vi "PXIe 4113 Config.vi"(8 "error in (no error)":errorcluster, 11 "Device Ref in":T1 format="%.0x") -> (0 "error out":errorcluster, 2 "instrument handle out":refnum<k15>, 3 "Device Ref out":T1 format="%.0x")   [LabVIEW 2015, in "PXIe 4113 Engine.lvlib"]
uses:
  PXIe 4113 Engine.lvlib
  <vilib>/NI Veristand/Custom Device API/Custom Device Item Ref.ctl
  <instrlib>/niDCPower/nidcpower.llb/niDCPower Source Mode.ctl
  <instrlib>/niDCPower/nidcpower.llb/niDCPower Output Function.ctl
  <instrlib>/niDCPower/nidcpower.llb/niDCPower Sense.ctl
  Shared/Constants.vi
  <vilib>/NI Veristand/Custom Device API/Get Item Property (String).vi
  <vilib>/NI Veristand/Custom Device API/Custom Device API.lvlib
  Shared/PXIe 4113 Shared.lvlib
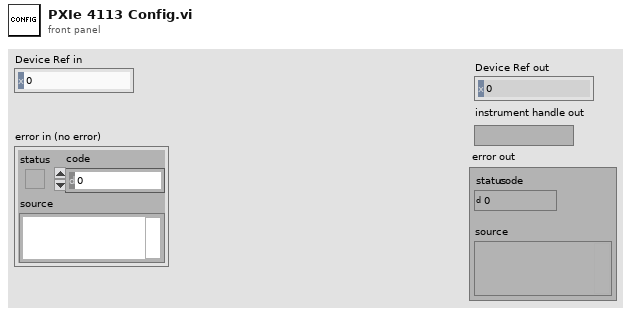
[diagram p1: front panel]
types:
  T1 = typedef "Custom Device API.lvlib/Custom Device Item Ref.ctl" = u64
  T2 = typedef "niDCPower Sense.ctl" = i32
  T3 = typedef "niDCPower Output Function.ctl" = i32
  T4 = typedef "niDCPower Source Mode.ctl" = i32
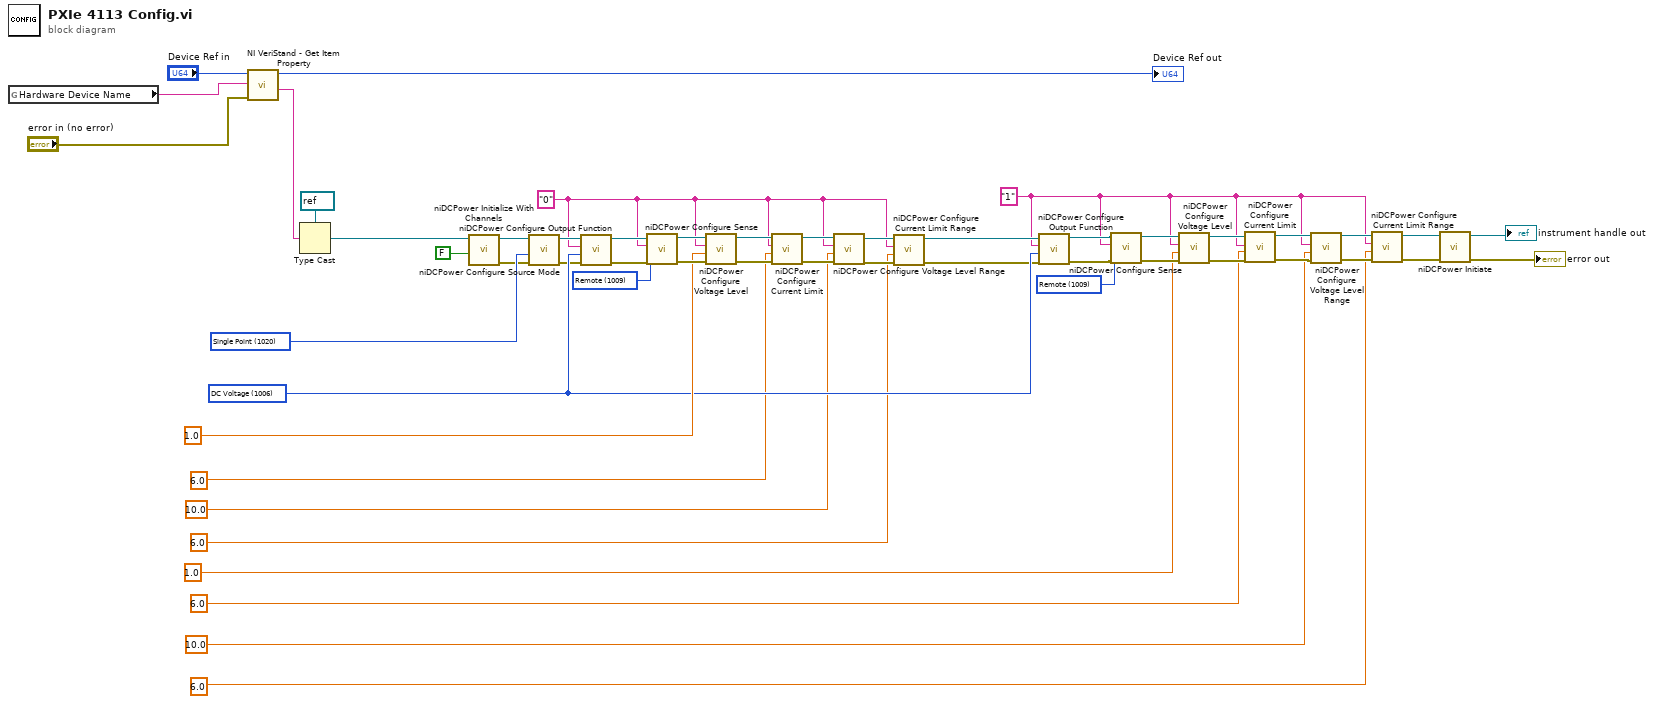
[diagram p0: block diagram]
diagram:
  w2 = T2 1009 items=["Local"=1008, "Remote"=1009] ("sense")
  w3 = T2 1009 items=["Local"=1008, "Remote"=1009] ("sense")
  w36 = T3 1006 items=["DC Voltage"=1006, "DC Current"=1007, "Pulse Voltage"=1049, "Pulse Current"=1050] ("output function")
  w38 = T4 1020 items=["Single Point"=1020, "Sequence"=1021] ("source mode")
  w19 = "1" ("channel name")
  w26 = "0" ("channel name")
  n1 = global read "Constants.vi" "Hardware Device Name"() -> (w34:string)
  n2 = call-poly <vilib>:"NI VeriStand - Get Item Property.vi"("error in (no error)"="error in (no error)", "Property Name"=w34, "Item Ref in"="Device Ref in") -> ("Value"=w6:string, "Item Ref out"=→"Device Ref out":T1)  [unwired: 5 in, 2 out]
  n3 = Type Cast(type=refnum<k15> refnum ("resource name"), x=w6) -> (*(type *) &x=w4:refnum<k15>)
  n4 = call <instrlib>:"niDCPower Initialize With Channels.vi"("reset (false)"=FALSE, "resource name"=w4) -> ("error out"=w11:errorcluster, "instrument handle out"=w52:refnum<k15>)  [unwired: 8 in]
  n5 = call <instrlib>:"niDCPower Configure Source Mode.vi"("error in (no error)"=w11, "source mode"=w38, "instrument handle"=w52) -> ("error out"=w10:errorcluster, "instrument handle out"=w51:refnum<k15>)  [unwired: 7 in]
  n6 = call <instrlib>:"niDCPower Configure Output Function.vi"("error in (no error)"=w10, "output function"=w36, "channel name"=w26, "instrument handle"=w51) -> ("error out"=w47:errorcluster, "instrument handle out"=w48:refnum<k15>)  [unwired: 6 in]
  n7 = call <instrlib>:"niDCPower Configure Sense.vi"("error in (no error)"=w47, "sense"=w3, "channel name"=w26, "instrument handle"=w48) -> ("error out"=w50:errorcluster, "instrument handle out"=w49:refnum<k15>)  [unwired: 6 in]
  n8 = call <instrlib>:"niDCPower Configure Voltage Level.vi"("error in (no error)"=w50, "voltage level"=1.0, "channel name"=w26, "instrument handle"=w49) -> ("error out"=w45:errorcluster, "instrument handle out"=w46:refnum<k15>)  [unwired: 6 in]
  n9 = call <instrlib>:"niDCPower Configure Current Limit.vi"("error in (no error)"=w45, "current limit"=6.0, "channel name"=w26, "instrument handle"=w46) -> ("error out"=w29:errorcluster, "instrument handle out"=w30:refnum<k15>)  [unwired: 6 in]
  n10 = call <instrlib>:"niDCPower Configure Voltage Level Range.vi"("error in (no error)"=w29, "voltage level range"=10.0, "channel name"=w26, "instrument handle"=w30) -> ("error out"=w32:errorcluster, "instrument handle out"=w31:refnum<k15>)  [unwired: 6 in]
  n11 = call <instrlib>:"niDCPower Configure Current Limit Range.vi"("error in (no error)"=w32, "current limit range"=6.0, "channel name"=w26, "instrument handle"=w31) -> ("error out"=w27:errorcluster, "instrument handle out"=w28:refnum<k15>)  [unwired: 6 in]
  n12 = call <instrlib>:"niDCPower Configure Output Function.vi"("error in (no error)"=w27, "output function"=w36, "channel name"=w19, "instrument handle"=w28) -> ("error out"=w43:errorcluster, "instrument handle out"=w44:refnum<k15>)  [unwired: 6 in]
  n13 = call <instrlib>:"niDCPower Configure Sense.vi"("error in (no error)"=w43, "sense"=w2, "channel name"=w19, "instrument handle"=w44) -> ("error out"=w42:errorcluster, "instrument handle out"=w41:refnum<k15>)  [unwired: 6 in]
  n14 = call <instrlib>:"niDCPower Configure Voltage Level.vi"("error in (no error)"=w42, "voltage level"=1.0, "channel name"=w19, "instrument handle"=w41) -> ("error out"=w39:errorcluster, "instrument handle out"=w40:refnum<k15>)  [unwired: 6 in]
  n15 = call <instrlib>:"niDCPower Configure Current Limit.vi"("error in (no error)"=w39, "current limit"=6.0, "channel name"=w19, "instrument handle"=w40) -> ("error out"=w21:errorcluster, "instrument handle out"=w23:refnum<k15>)  [unwired: 6 in]
  n16 = call <instrlib>:"niDCPower Configure Voltage Level Range.vi"("error in (no error)"=w21, "voltage level range"=10.0, "channel name"=w19, "instrument handle"=w23) -> ("error out"=w25:errorcluster, "instrument handle out"=w24:refnum<k15>)  [unwired: 6 in]
  n17 = call <instrlib>:"niDCPower Configure Current Limit Range.vi"("error in (no error)"=w25, "current limit range"=6.0, "channel name"=w19, "instrument handle"=w24) -> ("error out"=w20:errorcluster, "instrument handle out"=w22:refnum<k15>)  [unwired: 6 in]
  n18 = call <instrlib>:"niDCPower Initiate.vi"("error in (no error)"=w20, "instrument handle"=w22) -> ("error out"=→"error out":errorcluster, "instrument handle out"=→"instrument handle out":refnum<k15>)  [unwired: 8 in]
